vi "For diagram.vi"(8 "Предыдущий массив":dbl[](array[numeric]), 9 "Номер импульса":i32, 11 "Время в милисикундах":i32) -> (0 "Кол-во точек (время в милисек)":i32[](array[numeric]), 1 "Номер импульса (0 или 1)":i32[](array[numeric]))   [LabVIEW 2012]
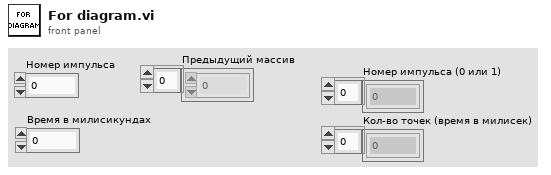
[diagram p1: front panel]
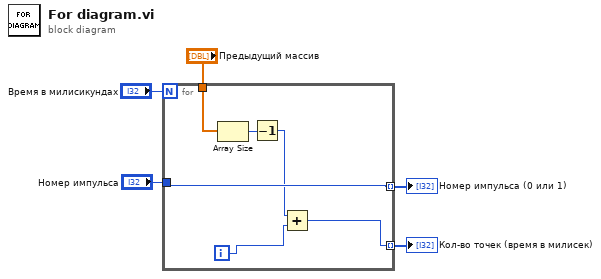
[diagram p0: block diagram]
diagram:
  n1 = for {
    N: "Время в милисикундах" -> [_]
    tunnel: [w11] -> w2 mode=indexing
    tunnel: [w8] -> w1 mode=indexing
    tunnel: "Номер импульса" -> [w11]
    tunnel: "Предыдущий массив" -> [w6]
    i -> [w9]
    n2 = Array Size(array=w6) -> (size(s)=w10:i32)
    n3 = Decrement(x=w10) -> (x-1=w7:i32)
    n4 = Add(x=w7, y=w9) -> (x+y=w8:i32)
  }
  "Номер импульса (0 или 1)" <- w2
  "Кол-во точек (время в милисек)" <- w1
